vi "SimulatedSweep.vi"(8 "error in (no error)":errorcluster, 11 "Map":T1) -> (0 "error out":errorcluster, 1 "Sweeps Valid":bool[](array[boolean]), 3 "map out":T1, 4 "sweep times":dbl[](array[numeric]), 5 "channels":string[](array[string]), 6 "current sweep frequencies":dbl[](array[numeric]))   [LabVIEW 2017, in "EmsaAcquisition.lvlib"]
uses:
  <vilib>/addons/InsightCM/Devices/Shared/Emsa/EmsaAcquisition/EmsaAcquisition.lvlib
  <vilib>/addons/PointValueMap/controls/PointMap.ctl
  <vilib>/addons/InsightCM/Devices/Shared/Emsa/EmsaAcquisition/subVIs/SimulatedConfigRefGlobal.vi
  <vilib>/addons/PointValueMap/PointValueMap.lvlib
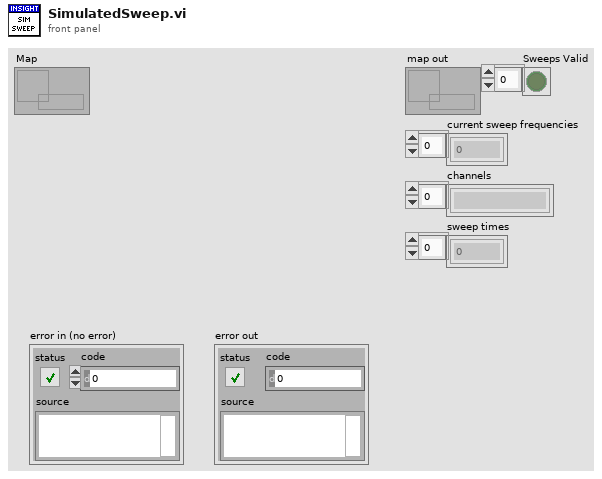
[diagram p1: front panel]
types:
  T1 = typedef "PointValueMap.lvlib/PointMap.ctl" = refnum<data-value>
  T2 = typedef "EmsaAcquisition.lvlib/SimulatedConfigRefs.ctl" = cluster{"SimulatedSignalConfig":refnum<vi>}
  T3 = typedef "EmsaAcquisition.lvlib/SimulatedSignalConfig.ctl" = cluster{"Channel Name":string[], "Valid":bool[], "Hardware Channel":string[], "Unit":string[], "Sweep Configs":T4[]}
  T4 = typedef "EmsaAcquisition.lvlib/SimulatedSweepConfig.ctl" = cluster{"Sweep Frequency List":cluster{"frequency":dbl, "bandwidth":dbl}[], "Detection Time":dbl, "Detection Mode":enum16{"Peak", "Quasi Peak", "Average"}, "Full Scale Volts":dbl, "Total Sweep Pts":i32, "Sweep Pointer":i32, "Sweep":T5[], "Sweep Start Time":timestamp}
  T5 = typedef "EmsaAcquisition.lvlib/SweepElement.ctl" = cluster{"Frequency":dbl, "Amplitude":dbl}
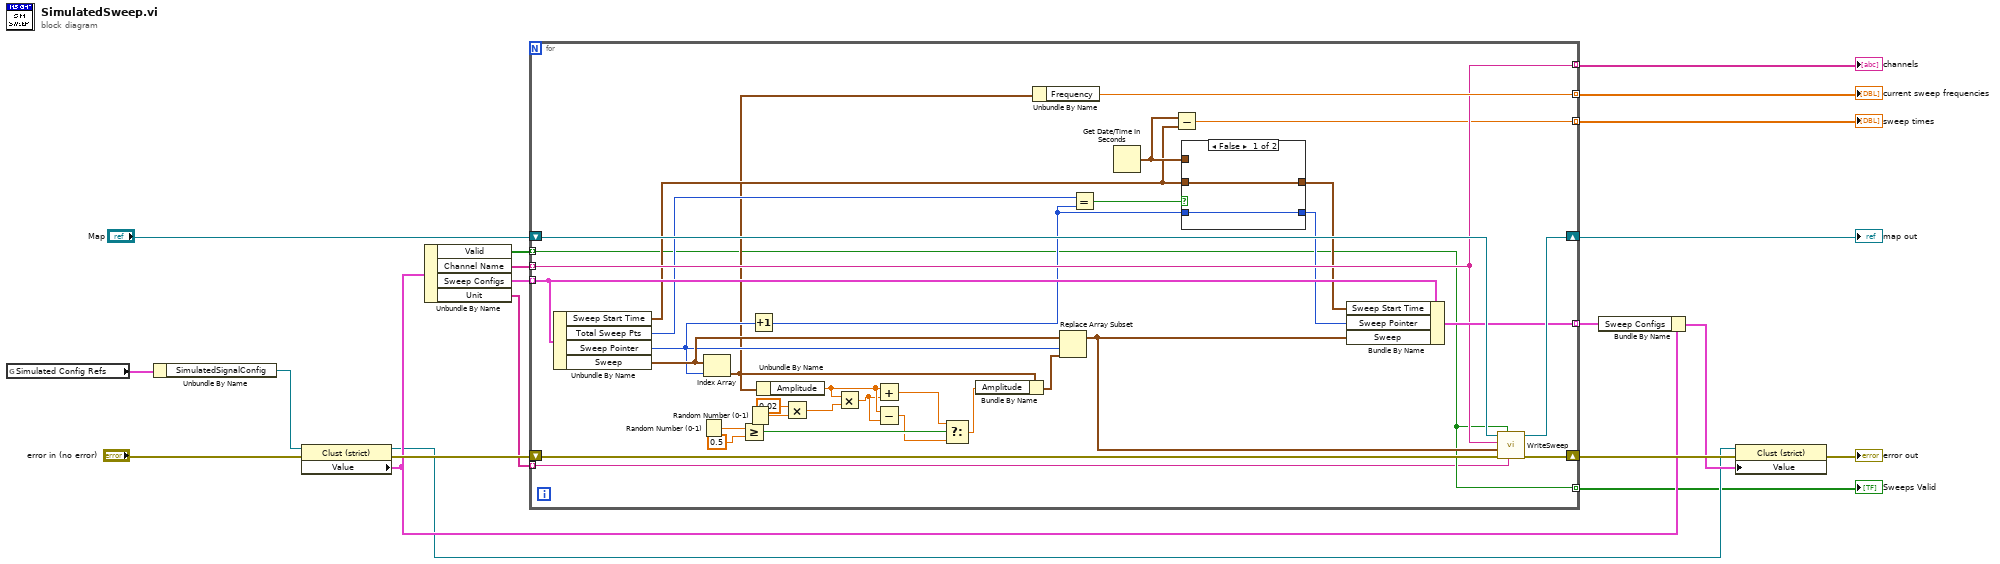
[diagram p0: block diagram]
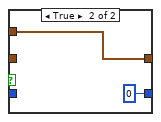
[diagram p2: hidden frame]
diagram:
  n1 = global read "SimulatedConfigRefGlobal.vi" "Simulated Config Refs"() -> (w20:T2)
  n2 = Unbundle By Name(w20) -> ("SimulatedSignalConfig"=w19:refnum<vi>)
  n3 = property class="Clust (strict)"(reference=w19, error in="error in (no error)") -> (reference out=w7:refnum<vi>, error out=w17:errorcluster, "Value"=w10:T3)
  n4 = Unbundle By Name(w10) -> ("Valid"=w12:bool[], "Channel Name"=w16:string[], "Sweep Configs"=w15:T4[], "Unit"=w1:string[])
  n5 = for {
    shift-right: [w53] -> w11
    shift-left: w17 -> [w54]
    tunnel: [w22] -> w5 mode=indexing
    tunnel: w16 -> [w43] mode=indexing
    tunnel: w15 -> [w48] mode=indexing
    shift-right: [w51] -> w13
    shift-left: "Map" -> [w52]
    tunnel: w12 -> [w22] mode=indexing
    tunnel: [w45] -> w9 mode=indexing
    tunnel: [w44] -> w4 mode=indexing
    tunnel: [w43] -> w3 mode=indexing
    tunnel: [w35] -> w2 mode=indexing
    tunnel: w1 -> [w21] mode=indexing
    n6 = Unbundle By Name(w48) -> ("Sweep Start Time"=w36:timestamp, "Total Sweep Pts"=w42:i32, "Sweep Pointer"=w46:i32, "Sweep"=w50:T5[])
    n7 = Random Number (0-1)() -> (number: 0 to 1=w33:dbl)
    n8 = Index Array(array=w50, index=w46) -> (element=w34:T5)
    n9 = Greater Or Equal?(x=w33, y=0.5) -> (x >= y?=w31:bool)
    n10 = Random Number (0-1)() -> (number: 0 to 1=w25:dbl)
    n11 = Increment(x=w46) -> (x+1=w40:i32)
    n12 = Unbundle By Name(w34) -> ("Amplitude"=w28:dbl)
    n13 = Multiply(x=0.02, y=w25) -> (x*y=w23:dbl)
    n14 = Multiply(x=w28, y=w23) -> (x*y=w27:dbl)
    n15 = Add(x=w28, y=w27) -> (x+y=w30:dbl)
    n16 = Subtract(x=w28, y=w27) -> (x-y=w26:dbl)
    n17 = Select(t=w30, s=w31, f=w26) -> (s? t:f=w29:dbl)
    n18 = Bundle By Name(cluster=w34, "Amplitude"=w29) -> (w49:T5)
    n19 = Unbundle By Name(w34) -> ("Frequency"=w44:dbl)
    n20 = Replace Array Subset(array=w50, new element=w49, index=w46) -> (w47:T5[])
    n21 = Equal?(x=w42, y=w40) -> (x = y?=w41:bool)
    n22 = Get Date/Time In Seconds() -> (seconds since 1Jan1904=w37:timestamp)
    n23 = Subtract(x=w37, y=w36) -> (x-y=w35:dbl)
    n24 = case shown="False" w41 {
      tunnel: [w56 0] -> w39
      tunnel: w40 -> [w56 _]
      tunnel: w36 -> [w55 _]
      tunnel: [w55 w57] -> w38
      tunnel: w37 -> [_ w57]
      frame False {
      }
      frame True {
      }
    }
    n25 = Bundle By Name(cluster=w48, "Sweep Start Time"=w38, "Sweep Pointer"=w39, "Sweep"=w47) -> (w45:T4)
    n26 = call <vilib>:"WriteSweep.vi"("unit"=w21, "sweep valid"=w22, "error in (no error)"=w54, "sweep"=w47, "channel"=w43, "map"=w52) -> ("error out"=w53:errorcluster, "map out"=w51:T1)  [unwired: 4 in]
  }
  "map out" <- w13
  "Sweeps Valid" <- w5
  "current sweep frequencies" <- w4
  "channels" <- w3
  "sweep times" <- w2
  n27 = Bundle By Name(cluster=w10, "Sweep Configs"=w9) -> (w8:T3)
  n28 = property class="Clust (strict)"(reference=w7, error in=w11, "Value"=w8) -> (error out=→"error out":errorcluster)  [unwired: 1 out]
